vi "Get Display Name.vi"(8 "error in (no error)":errorcluster, 11 "ClickableText in":refnum<class "ClickableText.lvclass">) -> (0 "error out":errorcluster, 2 "localized name":string, 3 "ClickableText out":refnum<class "ClickableText.lvclass">)   [LabVIEW 2009, in "NavScreen.lvlib" / "ClickableText.lvclass"]
uses:
  ClickableText.lvclass
  ClickableText.lvclass/ClickableText.ctl
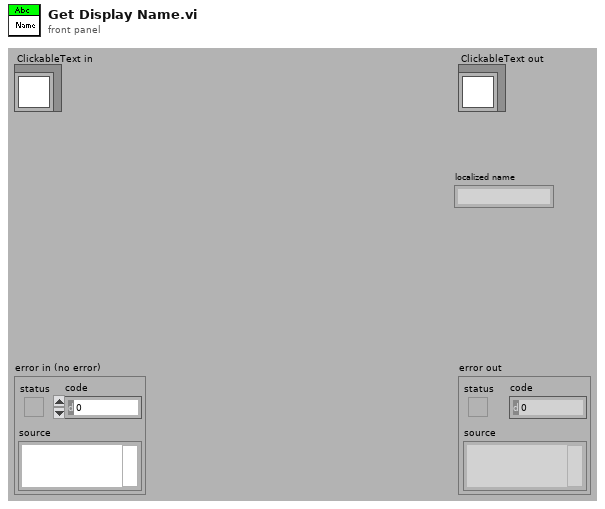
[diagram p1: front panel]
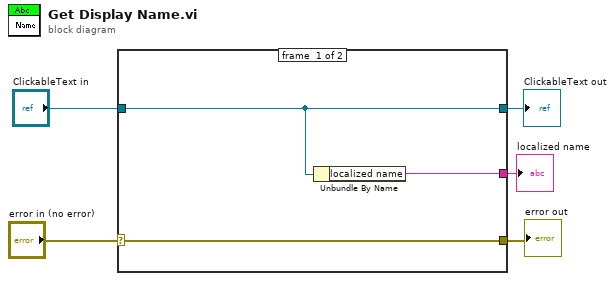
[diagram p0: block diagram]
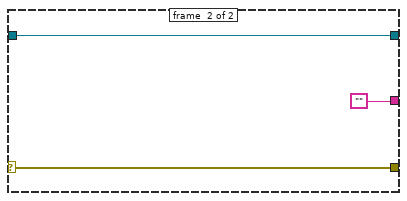
[diagram p2: hidden frame]
diagram:
  n1 = case shown="No Error" "error in (no error)" {
    selector: "error in (no error)" -> [w8 w11]
    tunnel: [w8 w11] -> w4
    tunnel: [w7 w10] -> w2
    tunnel: "ClickableText in" -> [w7 w10]
    tunnel: [w6 ""] -> w1
    frame #0 {
      n2 = Unbundle By Name(w7) -> ("localized name"=w6:string)
    }
    frame #1 {
    }
  }
  "error out" <- w4
  "ClickableText out" <- w2
  "localized name" <- w1
